vi "get image array.vi"(8 "error in (no error)":errorcluster, 11 "Thorcam in":refnum<class "Thorcam.lvclass">) -> (0 "error out":errorcluster, 3 "Thorcam out":refnum<class "Thorcam.lvclass">)   [LabVIEW 2012, in "Thorcam.lvclass"]
uses:
  Thorcam.lvclass
  Thorcam.lvclass/Thorcam.ctl
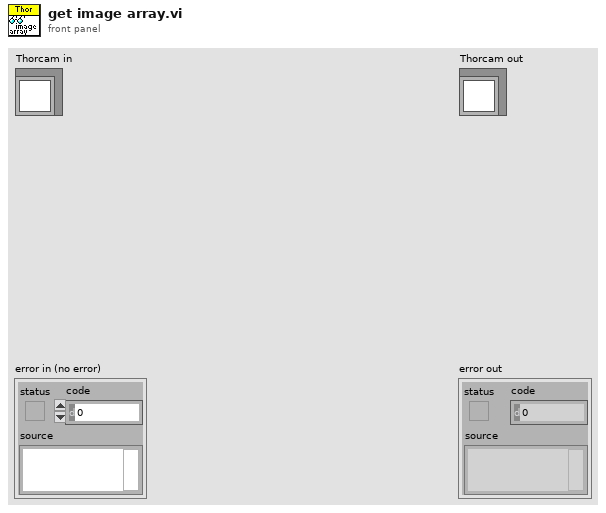
[diagram p1: front panel]
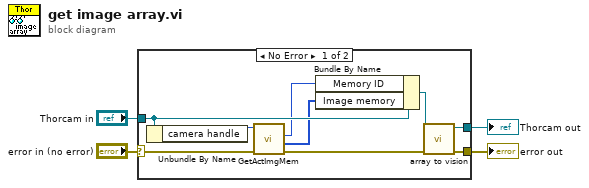
[diagram p0: block diagram]
diagram:
  n1 = case shown="No Error" "error in (no error)" {
    selector: "error in (no error)" -> [w12 w15]
    tunnel: [w7 w15] -> w3
    tunnel: [w5 w14] -> w1
    tunnel: "Thorcam in" -> [w11 w14]
    frame No Error {
      n2 = Unbundle By Name(w11) -> ("camera handle"=w13:u32)
      n3 = call <instrlib>:"GetActImgMem.vi"("error in"=w12, "Camera Handle In"=w13) -> ("error out"=w8:errorcluster, "Image Memory Out"=w9:u8[], "Memory Number"=w10:i32)  [unwired: 6 in, 1 out]
      n4 = Bundle By Name(cluster=w11, "Memory ID"=w10, "Image memory"=w9) -> (w6:refnum<class "Thorcam.lvclass">)
      n5 = call-dynamic "array to vision.vi"("error in (no error)"=w8, "Thorcam in"=w6) -> ("error out"=w7:errorcluster, "Thorcam out"=w5:refnum<class "Thorcam.lvclass">)  [unwired: 8 in]
    }
    frame Error {
    }
  }
  "error out" <- w3
  "Thorcam out" <- w1
